vi "Process Trainer PID.vi"() -> ()   [LabVIEW 2019]
uses:
  <vilib>/Modbus/slave/Create Slave Instance (TCP).vi
  <vilib>/addons/control/pid/pid.llb/PID (DBL).vi
  <vilib>/Modbus/slave/Modbus Slave.lvclass
  <vilib>/addons/control/pid/NI_PID_pid.lvlib
panel:
  out "x+1":dbl
  out "FV2 2":sgl
  out "appended array":dbl[](array[numeric])
  out "output":sgl
  in  "Flow Setpoint":dbl format="%.2f"
  out "Waveform Graph":sgl[](graph)
  in  "PID gains":T1={"proportional gain (Kc)"=1.0, "integral time (Ti, min)"=0.01, "derivative time (Td, min)"=0.0} {"derivative time (Td, min)" format="%.3f"; "integral time (Ti, min)" format="%.3f"; "proportional gain (Kc)" format="%.3f"}
  out "Numeric 7":sgl
  out "Numeric 6":sgl
  out "Numeric 5":sgl
  out "Numeric 4":sgl
  out "Numeric 3":sgl
  out "Numeric 2":sgl
  out "Numeric":sgl
  in  "Hot Water Setpoint":sgl(slide) scale=0.0..100.0
  in  "FV4":sgl(slide) scale=0.0..100.0
  in  "FV3":sgl(slide) scale=0.0..100.0
  in  "FV2":sgl(slide) scale=0.0..100.0
  in  "FV1":sgl(slide) scale=0.0..100.0
  in  "M2":sgl(slide) scale=0.0..100.0
  out "Hot Water Temp":sgl(knob) scale=0.0..100.0
  out "L1":sgl(knob) scale=0.0..100.0
  out "F2":sgl(knob) scale=0.0..100.0
  out "F1":sgl(knob) scale=0.0..100.0
  out "T3":sgl(knob) scale=0.0..100.0
  out "T2":sgl(knob) scale=0.0..100.0
  in  "stop":bool
  in  "M1":sgl(slide) scale=0.0..100.0
  out "T1":sgl(knob) scale=0.0..100.0
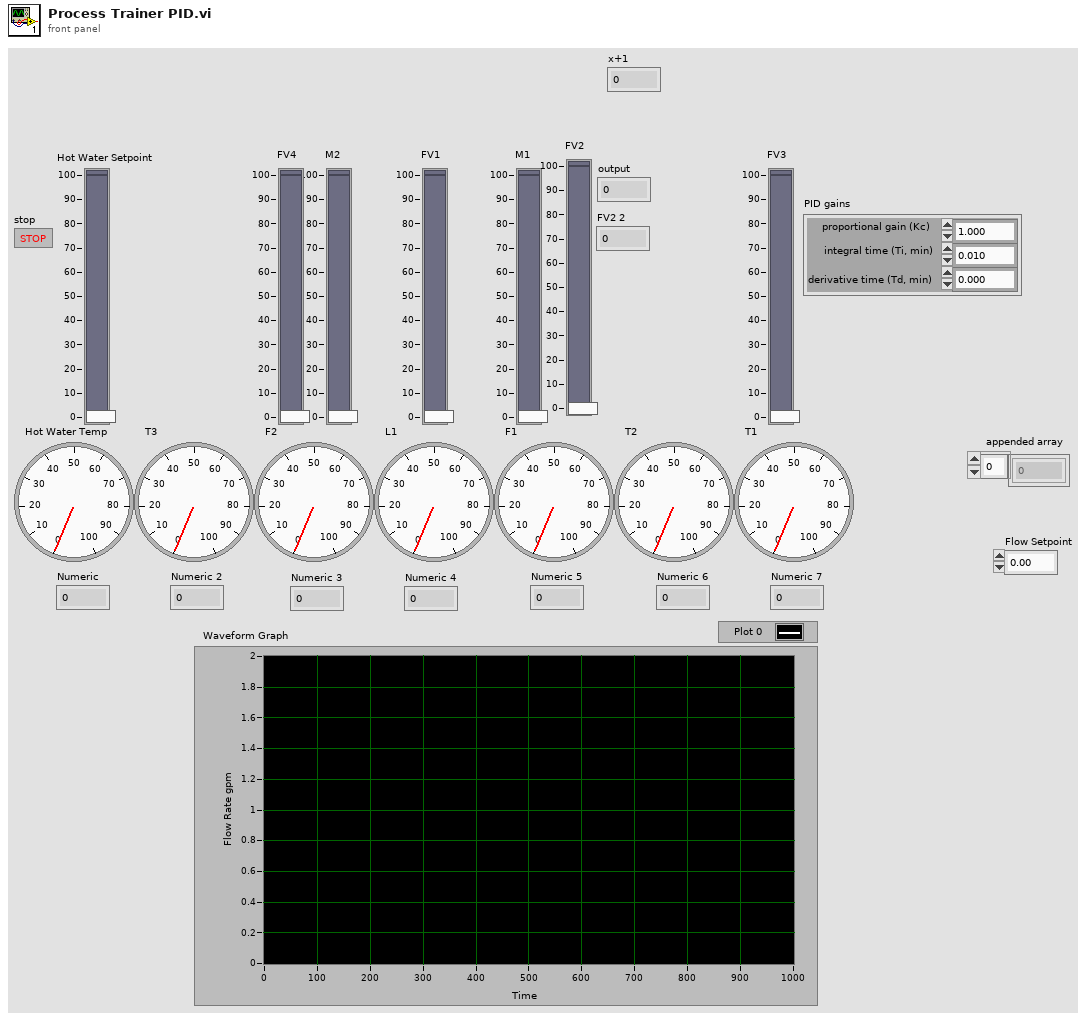
[diagram p1: front panel]
types:
  T1 = cluster{"proportional gain (Kc)":dbl, "integral time (Ti, min)":dbl, "derivative time (Td, min)":dbl}
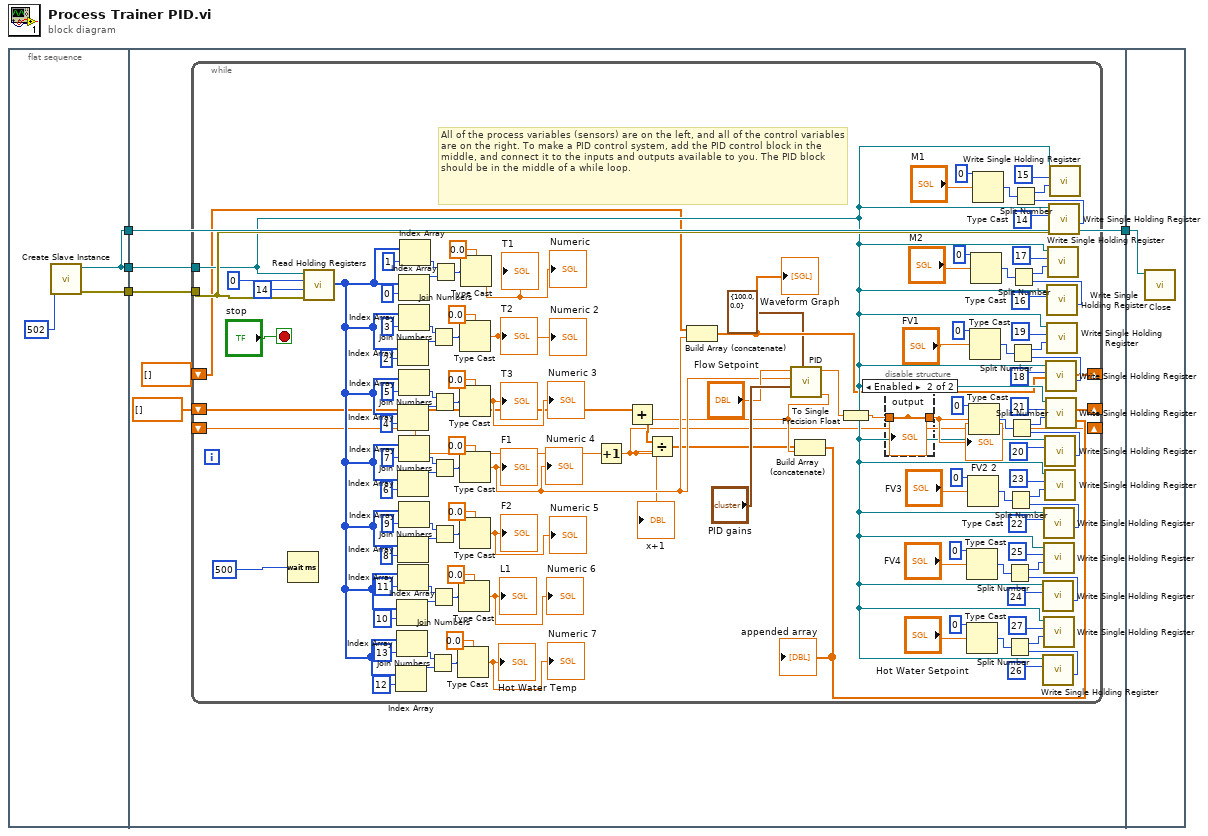
[diagram p0: block diagram]
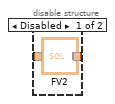
[diagram p2: hidden frame]
diagram:
  n1 = flat-sequence {
    tunnel: [w5] -> w4
    tunnel: [w6] -> w3
    tunnel: [w5] -> w2
    tunnel: w4 -> [w12]
    tunnel: w3 -> [w11]
    tunnel: [w10] -> w1
    tunnel: w2 -> [w10]
    tunnel: w1 -> [w134]
    frame #0 {
      n2 = call-poly <vilib>:"Create Slave Instance.vi"("port (502)"=u16 502) -> ("error out"=w6:errorcluster, "TCP slave instance"=w5:refnum<class "Modbus Slave.lvclass">)  [unwired: 9 in]
    }
    frame #1 {
      n3 = while {
        tunnel: w12 -> [w36]
        tunnel: w11 -> [w127]
        shift-right: [w26] -> _
        shift-left: sgl[] [] -> [w27]
        shift-right: [w23] -> _
        shift-left: dbl[] [] -> [w15]
        shift-right: [w13] -> _
        shift-left: _ -> [w14]
        stop <- "stop" stop-if-true
        # "All of the process variables (sensors) are on the left, and all of the control variables are on the right. To make a PID control system, add the PID control block in the middle, and connect it to the inputs and outputs available to you. The PID block should be in the middle of a while loop."
        n4 = Wait (ms)(milliseconds to wait=u32 500) -> ()  [unwired: 1 out]
        n5 = call-dynamic "Read Holding Registers.vi"("error in (no error)"=w127, "number of holding registers"=u16 14, "starting address"=u16 0, "Modbus slave in"=w36) -> ("register values"=w78:u16[])  [unwired: 5 in, 2 out]
        n6 = Index Array(array=w78, index=12) -> (element=w80:u16)
        n7 = Index Array(array=w78, index=10) -> (element=w86:u16)
        n8 = Index Array(array=w78, index=13) -> (element=w79:u16)
        n9 = Index Array(array=w78, index=2) -> (element=w110:u16)
        n10 = Index Array(array=w78, index=4) -> (element=w104:u16)
        n11 = Index Array(array=w78, index=6) -> (element=w98:u16)
        n12 = Index Array(array=w78, index=8) -> (element=w92:u16)
        n13 = Index Array(array=w78, index=11) -> (element=w85:u16)
        n14 = Index Array(array=w78, index=0) -> (element=w116:u16)
        n15 = Index Array(array=w78, index=3) -> (element=w109:u16)
        n16 = Index Array(array=w78, index=5) -> (element=w103:u16)
        n17 = Index Array(array=w78, index=7) -> (element=w97:u16)
        n18 = Index Array(array=w78, index=9) -> (element=w91:u16)
        n19 = Index Array(array=w78, index=1) -> (element=w115:u16)
        n20 = Join Numbers(hi=w79, lo=w80) -> ((hi.lo)=w81:u32)
        n21 = Join Numbers(hi=w109, lo=w110) -> ((hi.lo)=w111:u32)
        n22 = Join Numbers(hi=w85, lo=w86) -> ((hi.lo)=w87:u32)
        n23 = Join Numbers(hi=w103, lo=w104) -> ((hi.lo)=w105:u32)
        n24 = Join Numbers(hi=w97, lo=w98) -> ((hi.lo)=w99:u32)
        n25 = Join Numbers(hi=w91, lo=w92) -> ((hi.lo)=w93:u32)
        n26 = Join Numbers(hi=w115, lo=w116) -> ((hi.lo)=w117:u32)
        n27 = Type Cast(type=sgl 0.0, x=w81) -> (*(type *) &x=→"Hot Water Temp" →"Numeric 7":sgl)
        n28 = Type Cast(type=sgl 0.0, x=w87) -> (*(type *) &x=→"L1" →"Numeric 6":sgl)
        n29 = Type Cast(type=sgl 0.0, x=w111) -> (*(type *) &x=→"T2" →"Numeric 2":sgl)
        n30 = Type Cast(type=sgl 0.0, x=w105) -> (*(type *) &x=→"T3" →"Numeric 3":sgl)
        n31 = Type Cast(type=sgl 0.0, x=w99) -> (*(type *) &x=w19:sgl)
        "F1" <- w19
        "Numeric 4" <- w19
        n32 = Type Cast(type=sgl 0.0, x=w93) -> (*(type *) &x=→"F2" →"Numeric 5":sgl)
        n33 = Type Cast(type=sgl 0.0, x=w117) -> (*(type *) &x=→"T1" →"Numeric":sgl)
        n34 = Increment(x=w14) -> (x+1=w13:dbl)
        "x+1" <- w13
        n35 = Build Array (concatenate)(w27, w19) -> (w26:sgl[])
        "Waveform Graph" <- w26
        n36 = call-poly <vilib>:"PID.vi"("output range"=cluster{"output high":dbl, "output low":dbl} {"output high"=100.0, "output low"=0.0}, "PID gains"="PID gains", "process variable"=w19, "setpoint"="Flow Setpoint") -> ("dt out (s)"=w18:dbl, "output"=w22:dbl)  [unwired: 6 in]
        n37 = Add(x=w15, y=w18) -> (x+y=w17:dbl[])
        n38 = Divide(x=w17, y=w13) -> (x/y=w16:dbl[])
        n39 = Build Array (concatenate)(w16, w18) -> (w23:dbl[])
        "appended array" <- w23
        n40 = To Single Precision Float(number=w22) -> (single precision float=w21:sgl)
        n41 = disable-structure shown="Enabled" {
          disable-tunnel: ["FV2" w133] -> w58
          disable-tunnel: w21 -> [_ w133]
          frame Disabled {
          }
          frame Enabled {
            "output" <- w133
          }
        }
        "FV2 2" <- w58
        n42 = Type Cast(type=u32 0, x="FV4") -> (*(type *) &x=w46:u32)
        n43 = Type Cast(type=u32 0, x="Hot Water Setpoint") -> (*(type *) &x=w39:u32)
        n44 = Type Cast(type=u32 0, x="FV3") -> (*(type *) &x=w53:u32)
        n45 = Type Cast(type=u32 0, x=w58) -> (*(type *) &x=w60:u32)
        n46 = Type Cast(type=u32 0, x="FV1") -> (*(type *) &x=w66:u32)
        n47 = Type Cast(type=u32 0, x="M2") -> (*(type *) &x=w73:u32)
        n48 = Type Cast(type=u32 0, x="M1") -> (*(type *) &x=w123:u32)
        n49 = Split Number(x=w46) -> (hi(x)=w48:u16, lo(x)=w47:u16)
        n50 = Split Number(x=w39) -> (hi(x)=w41:u16, lo(x)=w40:u16)
        n51 = Split Number(x=w53) -> (hi(x)=w55:u16, lo(x)=w54:u16)
        n52 = Split Number(x=w60) -> (hi(x)=w62:u16, lo(x)=w61:u16)
        n53 = Split Number(x=w66) -> (hi(x)=w68:u16, lo(x)=w67:u16)
        n54 = Split Number(x=w73) -> (hi(x)=w75:u16, lo(x)=w74:u16)
        n55 = Split Number(x=w123) -> (hi(x)=w125:u16, lo(x)=w124:u16)
        n56 = call-dynamic "Write Single Holding Register.vi"("holding register value"=w47, "address"=u16 24, "Modbus slave in"=w36) -> ()  [unwired: 7 in, 2 out]
        n57 = call-dynamic "Write Single Holding Register.vi"("holding register value"=w40, "address"=u16 26, "Modbus slave in"=w36) -> ()  [unwired: 7 in, 2 out]
        n58 = call-dynamic "Write Single Holding Register.vi"("holding register value"=w54, "address"=u16 22, "Modbus slave in"=w36) -> ()  [unwired: 7 in, 2 out]
        n59 = call-dynamic "Write Single Holding Register.vi"("holding register value"=w48, "address"=u16 25, "Modbus slave in"=w36) -> ()  [unwired: 7 in, 2 out]
        n60 = call-dynamic "Write Single Holding Register.vi"("holding register value"=w41, "address"=u16 27, "Modbus slave in"=w36) -> ()  [unwired: 7 in, 2 out]
        n61 = call-dynamic "Write Single Holding Register.vi"("holding register value"=w61, "address"=u16 20, "Modbus slave in"=w36) -> ()  [unwired: 7 in, 2 out]
        n62 = call-dynamic "Write Single Holding Register.vi"("holding register value"=w55, "address"=u16 23, "Modbus slave in"=w36) -> ()  [unwired: 7 in, 2 out]
        n63 = call-dynamic "Write Single Holding Register.vi"("holding register value"=w67, "address"=u16 18, "Modbus slave in"=w36) -> ()  [unwired: 7 in, 2 out]
        n64 = call-dynamic "Write Single Holding Register.vi"("holding register value"=w62, "address"=u16 21, "Modbus slave in"=w36) -> ()  [unwired: 7 in, 2 out]
        n65 = call-dynamic "Write Single Holding Register.vi"("holding register value"=w74, "address"=u16 16, "Modbus slave in"=w36) -> ()  [unwired: 7 in, 2 out]
        n66 = call-dynamic "Write Single Holding Register.vi"("holding register value"=w68, "address"=u16 19, "Modbus slave in"=w36) -> ()  [unwired: 7 in, 2 out]
        n67 = call-dynamic "Write Single Holding Register.vi"("holding register value"=w75, "address"=u16 17, "Modbus slave in"=w36) -> ()  [unwired: 7 in, 2 out]
        n68 = call-dynamic "Write Single Holding Register.vi"("error in (no error)"=w127, "holding register value"=w124, "address"=u16 14, "Modbus slave in"=w36) -> ()  [unwired: 6 in, 2 out]
        n69 = call-dynamic "Write Single Holding Register.vi"("holding register value"=w125, "address"=u16 15, "Modbus slave in"=w36) -> ()  [unwired: 7 in, 2 out]
      }
    }
    frame #2 {
      n70 = call-dynamic "Close.vi"("Modbus slave in"=w134) -> ()  [unwired: 10 in, 1 out]
    }
  }
